vi "BuildClass.vi"(6 "ProjectPath":path, 7 "Parent":enum16{"None", "Interface", "Class"}(ring)=enum."Interface", 8 "error in (no error)":errorcluster, 9 "This Application":refnum<vi>, 10 "ParentRef":refnum<vi>, 11 "iClass in":refnum<class "iClass.lvclass">) -> (0 "error out":errorcluster, 3 "iClass out":refnum<class "iClass.lvclass">)   [LabVIEW 2020, in "Mermaid.lvlib" / "iClass.lvclass"]
uses:
  iClass.lvclass
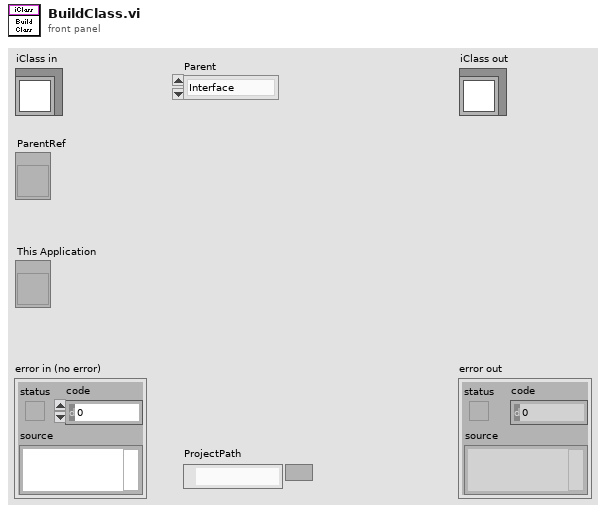
[diagram p1: front panel]
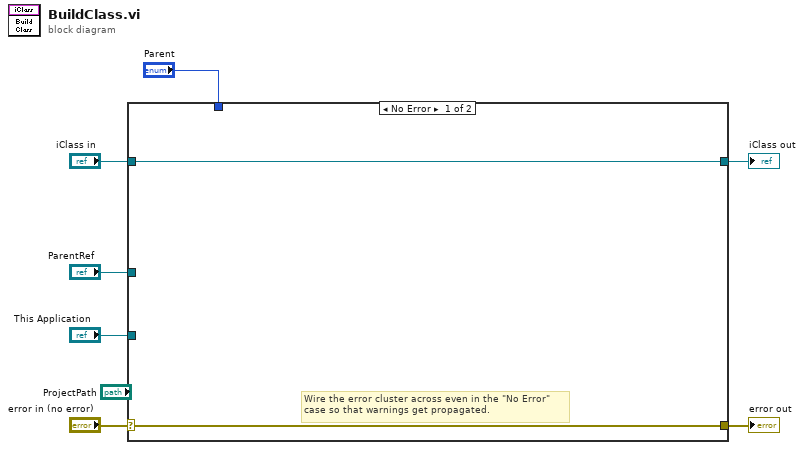
[diagram p0: block diagram]
diagram:
  n1 = case shown="No Error" "error in (no error)" {
    selector: "error in (no error)" -> [w8 w11]
    tunnel: [w8 w11] -> w6
    tunnel: [w9 w10] -> w4
    tunnel: "iClass in" -> [w9 w10]
    tunnel: "Parent" -> [_ _]
    tunnel: "ParentRef" -> [_ _]
    tunnel: "This Application" -> [_ _]
    frame No Error {
      # "Wire the error cluster across even in the \"No Error\"\ncase so that warnings get propagated."
    }
    frame Error {
    }
  }
  "error out" <- w6
  "iClass out" <- w4
